vi "__Get Path info for List.vi"(8 "error in (no error)":errorcluster, 11 "Path in":path) -> (0 "error out":errorcluster, 3 "Path info":string[](array[string]))   [LabVIEW 2011]
doc: "Parses the data associated with a local path to the format that is required to display it on the multicolumn listbox."
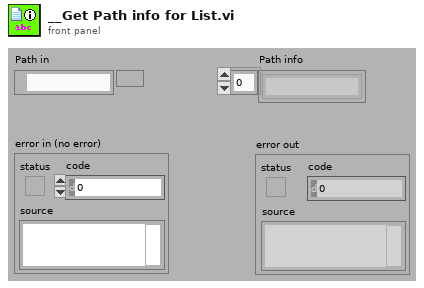
[diagram p1: front panel]
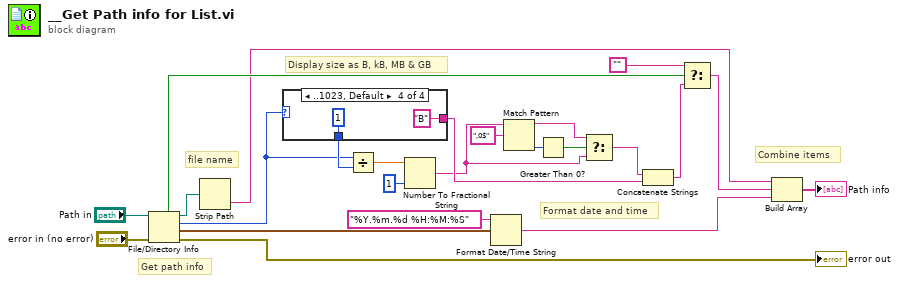
[diagram p0: block diagram]
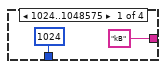
[diagram p2: hidden frame]
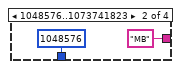
[diagram p3: hidden frame]
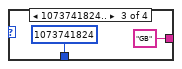
[diagram p4: hidden frame]
diagram:
  # "Combine items"
  # "Format date and time"
  # "Display size as B, kB, MB & GB"
  # "Get path info"
  # "file name"
  n1 = File/Directory Info(path="Path in", error in="error in (no error)") -> (path out=w2:path, directory=w16:bool, size=w12:i64, last mod=w21:timestamp, error out=→"error out":errorcluster)  [unwired: 2 out]
  n2 = Strip Path(path=w2) -> (name=w1:string)  [unwired: 1 out]
  n3 = case shown="..1023, Default" w12 {
    tunnel: [i64 1024 ("size") i64 1048576 ("size") i64 1073741824 ("size") i64 1 ("size")] -> w13
    tunnel: ["kB" ("string") "MB" ("string") "GB" ("string") "B" ("string")] -> w11
    frame 1024..1048575 {
    }
    frame 1048576..1073741823 {
    }
    frame 1073741824.. {
    }
    frame ..1023, Default {
    }
  }
  n4 = Divide(x=w12, y=w13) -> (x/y=w14:dbl)
  n5 = Number To Fractional String(number=w14, precision (6)=i16 1) -> (F-format string=w4:string)  [unwired: 2 in]
  n6 = Format Date/Time String(time format string (%c)="%Y.%m.%d %H:%M:%S", seconds (now)=w21) -> (date/time string=w20:string)  [unwired: 1 in]
  n7 = Match Pattern(string=w4, regular expression=",0$") -> (before substring=w5:string, offset past match=w7:i32)  [unwired: 1 in, 2 out]
  n8 = Greater Than 0?(x=w7) -> (x > 0?=w6:bool)
  n9 = Select(t=w5, s=w6, f=w4) -> (s? t:f=w3:string)
  n10 = Concatenate Strings(w3, w11) -> (w10:string)
  n11 = Select(t="", s=w16, f=w10) -> (s? t:f=w17:string)
  n12 = Build Array(w1, w17, w20) -> (→"Path info":string[])
